vi "CPU_Power_Spec_CDB.vi"(7 "window":u16(ring) items=["None "=0, "Hanning"=1, "Hamming"=2, "Blackman-Harris"=3, "Exact Blackman"=4, "Blackman"=5, "Flat Top"=6, "4 Term B-Harris "=7, "7 Term B-Harris"=8, "Low Sidelobe"=9, "Blackman Nuttall"=11], 11 "Signal":cdb[](array[numeric])) -> (3 "Spectrum (no Avg)":dbl[](array[numeric]))   [LabVIEW 2020]
uses:
  <vilib>/Analysis/2dsp.llb/Power Spectrum (CDB).vi
  <vilib>/Analysis/NI_AALPro.lvlib
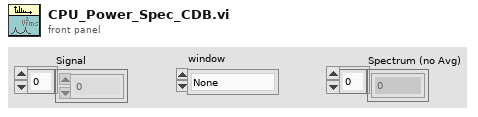
[diagram p1: front panel]
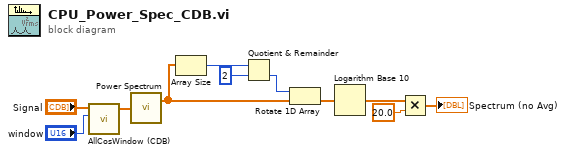
[diagram p0: block diagram]
diagram:
  n1 = call <vilib>:"AllCosWindow (CDB).vi"("window"="window", "X"="Signal") -> ("Windowed X"=w8:cdb[])  [unwired: 3 in, 1 out]
  n2 = call-poly <vilib>:"Power Spectrum.vi"("X"=w8) -> ("Power Spectrum"=w5:dbl[])  [unwired: 1 out]
  n3 = Array Size(array=w5) -> (size(s)=w4:i32)
  n4 = Quotient & Remainder(x=w4, y=2) -> (floor(x/y)=w1:i32)  [unwired: 1 out]
  n5 = Rotate 1D Array(1:w5, 2:w1) -> (0:w2:dbl[])
  n6 = Logarithm Base 10(1:w2) -> (0:w10:dbl[])
  n7 = Multiply(x=w10, y=sgl 20.0 ("dt")) -> (x*y=→"Spectrum (no Avg)":dbl[])
